vi "RunCL - Run All Tests.vi"(11 "Cmd Line Args":string[](array[string])=["C:\\BitBucket\\pipeline_test\\Source\\SampleLV.lvproj", "Main", "My Computer", "1234"]) -> (2 "Error Info":string, 3 "Error Code":i32)   [LabVIEW 2020]
uses:
  <userlib>/_OpenG.lib/file/file.llb/Append Path to Root if Relative - Scalar__ogtk.vi
  <vilib>/addons/_JKI Toolkits/Caraya/classes/Test Report.JUnit/Test Report.JUnit.lvclass
  <vilib>/addons/_JKI Toolkits/Caraya/classes/Test Runner/Test Runner.lvclass
  <vilib>/addons/_JKI Toolkits/Caraya/classes/Test Runner.Folder/Test Runner.Folder.lvclass
  <userlib>/_OpenG.lib/file/file.llb/File Exists - Scalar__ogtk.vi
panel:
  in  "Show Caraya GUI":bool=TRUE
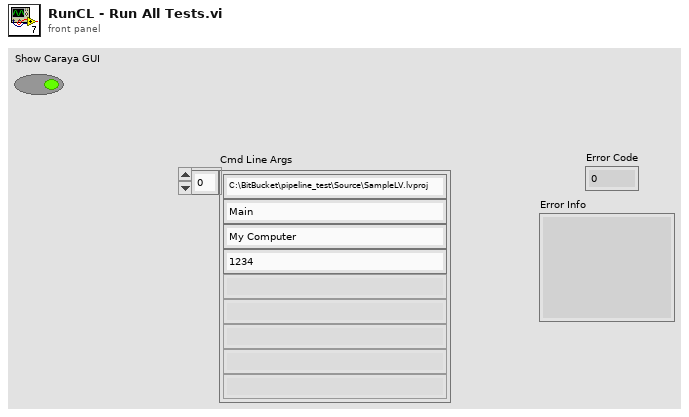
[diagram p1: front panel]
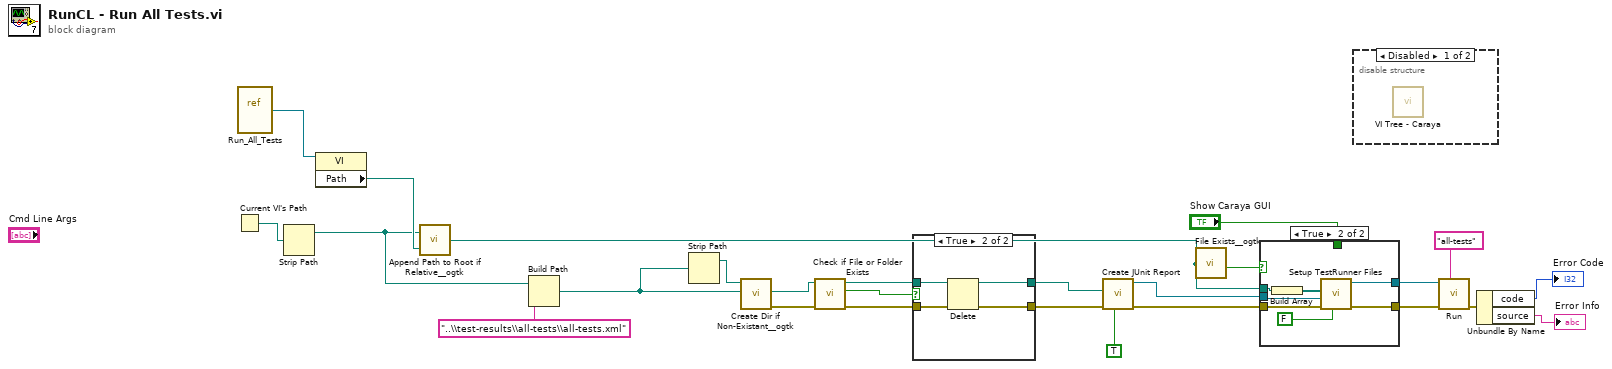
[diagram p0: block diagram]
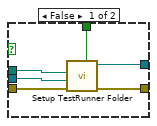
[diagram p3: hidden frame]
diagram:
  n1 = Current VI's Path() -> (path=w24:path)
  n2 = vi-ref "Run_All_Tests.vi"() -> (w25:refnum<vi>)
  n3 = Strip Path(path=w24) -> (stripped path=w4:path)  [unwired: 1 out]
  n4 = property class="VI"(reference=w25) -> ("Path"=w23:path)  [unwired: 1 in, 2 out]
  n5 = call-poly <userlib>:"Append Path to Root if Relative__ogtk.vi"("Absolute or Relative Path"=w23, "Root Path"=w4) -> ("Absolute or Appended Path"=w11:path)
  n6 = Build Path(base path=w4, name or relative path="..\\test-results\\all-tests\\all-tests.xml") -> (appended path=w20:path)
  n7 = Strip Path(path=w20) -> (stripped path=w21:path)  [unwired: 1 out]
  n8 = call <userlib>:"Create Dir if Non-Existant__ogtk.vi"("Directory Path"=w21) -> ("error out"=w7:errorcluster)  [unwired: 8 in, 2 out]
  n9 = call <vilib>:"Check if File or Folder Exists.vi"("error in (no error)"=w7, "path"=w20) -> ("error out"=w6:errorcluster, "file or folder exists?"=w19:bool, "dup path"=w18:path)  [unwired: 7 in]
  n10 = case shown="True" w19 {
    tunnel: w18 -> [w27 w31]
    tunnel: [w27 w30] -> w17
    tunnel: w6 -> [w26 w29]
    tunnel: [w26 w28] -> w5
    frame False {
    }
    frame True {
      n11 = Delete(path (use dialog)=w31, error in=w29) -> (deleted path=w30:path, error out=w28:errorcluster)  [unwired: 3 in, 1 out]
    }
  }
  n12 = call <vilib>:"Create JUnit Report.vi"("Verbose"=TRUE, "error in (no error)"=w5, "Report Path"=w17) -> ("error out"=w8:errorcluster, "Test Report.JUnit out"=w15:refnum<class "Test Report.JUnit.lvclass">)  [unwired: 7 in]
  n13 = call-poly <userlib>:"File Exists__ogtk.vi"("file path"=w11) -> ("exists"=w10:bool)  [unwired: 6 in, 1 out]
  n14 = case shown="True" w10 {
    tunnel: w15 -> [w37 w43]
    tunnel: [w36 w44] -> w14
    tunnel: "Show Caraya GUI" -> [w35 _]
    tunnel: w11 -> [w34 w41]
    tunnel: [w33 w39] -> w9
    tunnel: w8 -> [w32 w38]
    frame False {
      n15 = call <vilib>:"Setup TestRunner Folder.vi"("Interactive (T)"=w35, "error in (no error)"=w32, "Test Report"=w37, "Directory to search"=w34) -> ("error out"=w33:errorcluster, "Test Runner.Folder out"=w36:refnum<class "Test Runner.Folder.lvclass">)  [unwired: 6 in]
    }
    frame True {
      n16 = Build Array(w41) -> (w40:path[])
      n17 = call <vilib>:"Setup TestRunner Files.vi"("Inspect Recursively (T)"=FALSE, "error in (no error)"=w38, "Test Report"=w43, "Paths"=w40) -> ("error out"=w39:errorcluster, "Test Runner.Folder out"=w44:refnum<class "Test Runner.Folder.lvclass">)  [unwired: 6 in]
    }
  }
  n18 = disable-structure shown="Disabled" {
    frame Disabled {
      n19 = call <vilib>:"VI Tree - Caraya.vi"() -> ()  [unwired: 1 in]
    }
    frame Enabled {
    }
  }
  n20 = call <vilib>:"Run.vi"("Name"="all-tests", "error in (no error)"=w9, "Test Runner in"=w14) -> ("error out"=w3:errorcluster)  [unwired: 6 in, 2 out]
  n21 = Unbundle By Name(w3) -> ("code"=→"Error Code":i32, "source"=→"Error Info":string)
